vi "GaitDisplay.vi"() -> ()   [LabVIEW 2016]
uses:
  Classes/CAlex2-Display/CAlex2_Display.lvclass
  C:/Users/Rand/Documents/CAlex2-controller/Classes/CAlex2/CAlex2.lvclass
  C:/Users/Rand/Documents/CAlex2-controller/Classes/SerialChain/SerialChain.lvclass
  Classes/CAlex2/TypeDef/LowerBodyDim.ctl
  Classes/CAlex2/CAlex2.lvclass
  Classes/SerialChain/SerialChain.lvclass
panel:
  in  "port or service name":u16=11003
  in  "name":string="192.168.1.192"
  in  "Target":bool
  in  "Stop Button":bool
  in  "XY":bool
  in  "Reset":bool
  in  "Leg Position":refnum<k7>(container)
  # "Up"
  # "Back"
  # "Front"
  # "Down"
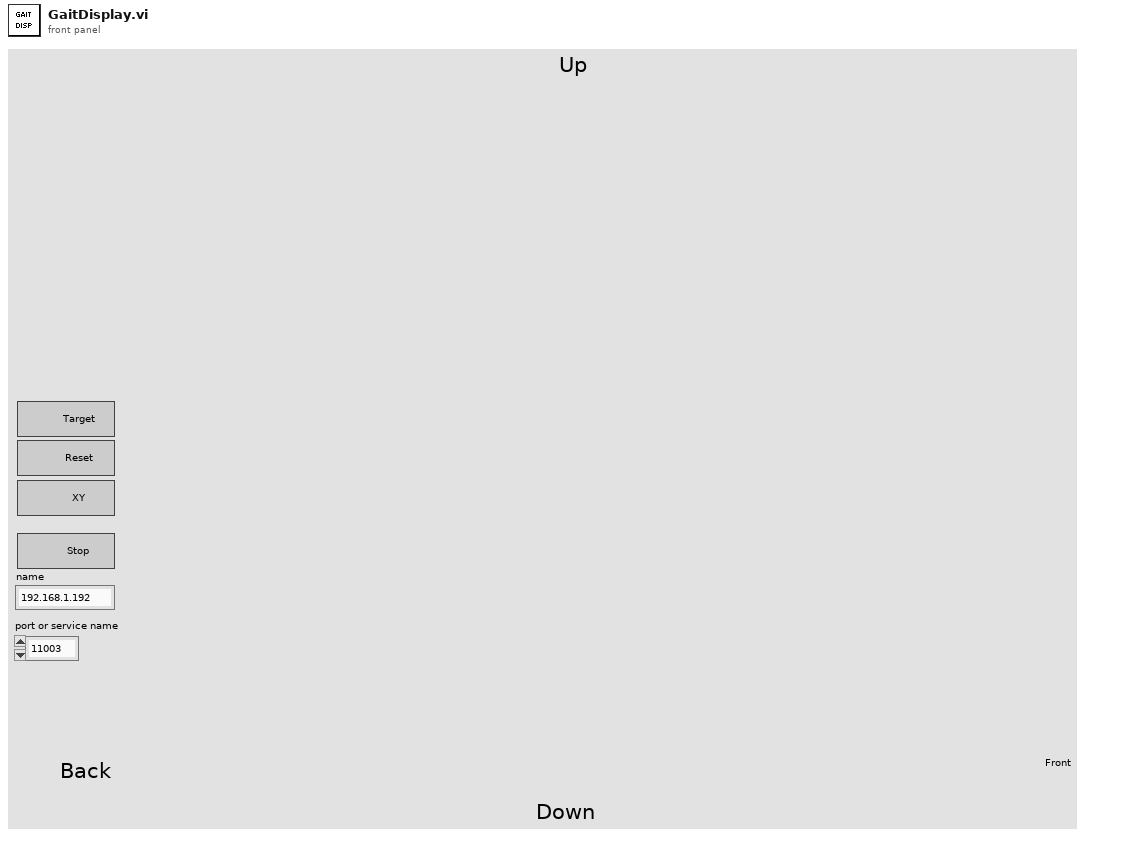
[diagram p1: front panel]
types:
  T1 = enum16{"big-endian, network order", "native, host order", "little-endian"}
  T2 = cluster{"AxisLabel":string[], "AxisMax":dbl[], "AxisMin":dbl[]}
  T3 = typedef "CAlex2.lvclass/LowerBodyDim.ctl" = cluster{"BodyDim":cluster{"ThighLt (m)":dbl, "ShankLt (m)":dbl, "HipWd (m)":dbl}, "BodyWt":cluster{"Thigh (kg)":dbl, "Shank (kg)":dbl}, "Cuff Loc":cluster{"HipCuffWd (m)":dbl, "HipCuffHt (m)":dbl, "HipFwdShift (m)":dbl, "ThighToKnee (m)":dbl, "ThighCuffDist (m)":dbl, "ShankToKnee (m)":dbl}}
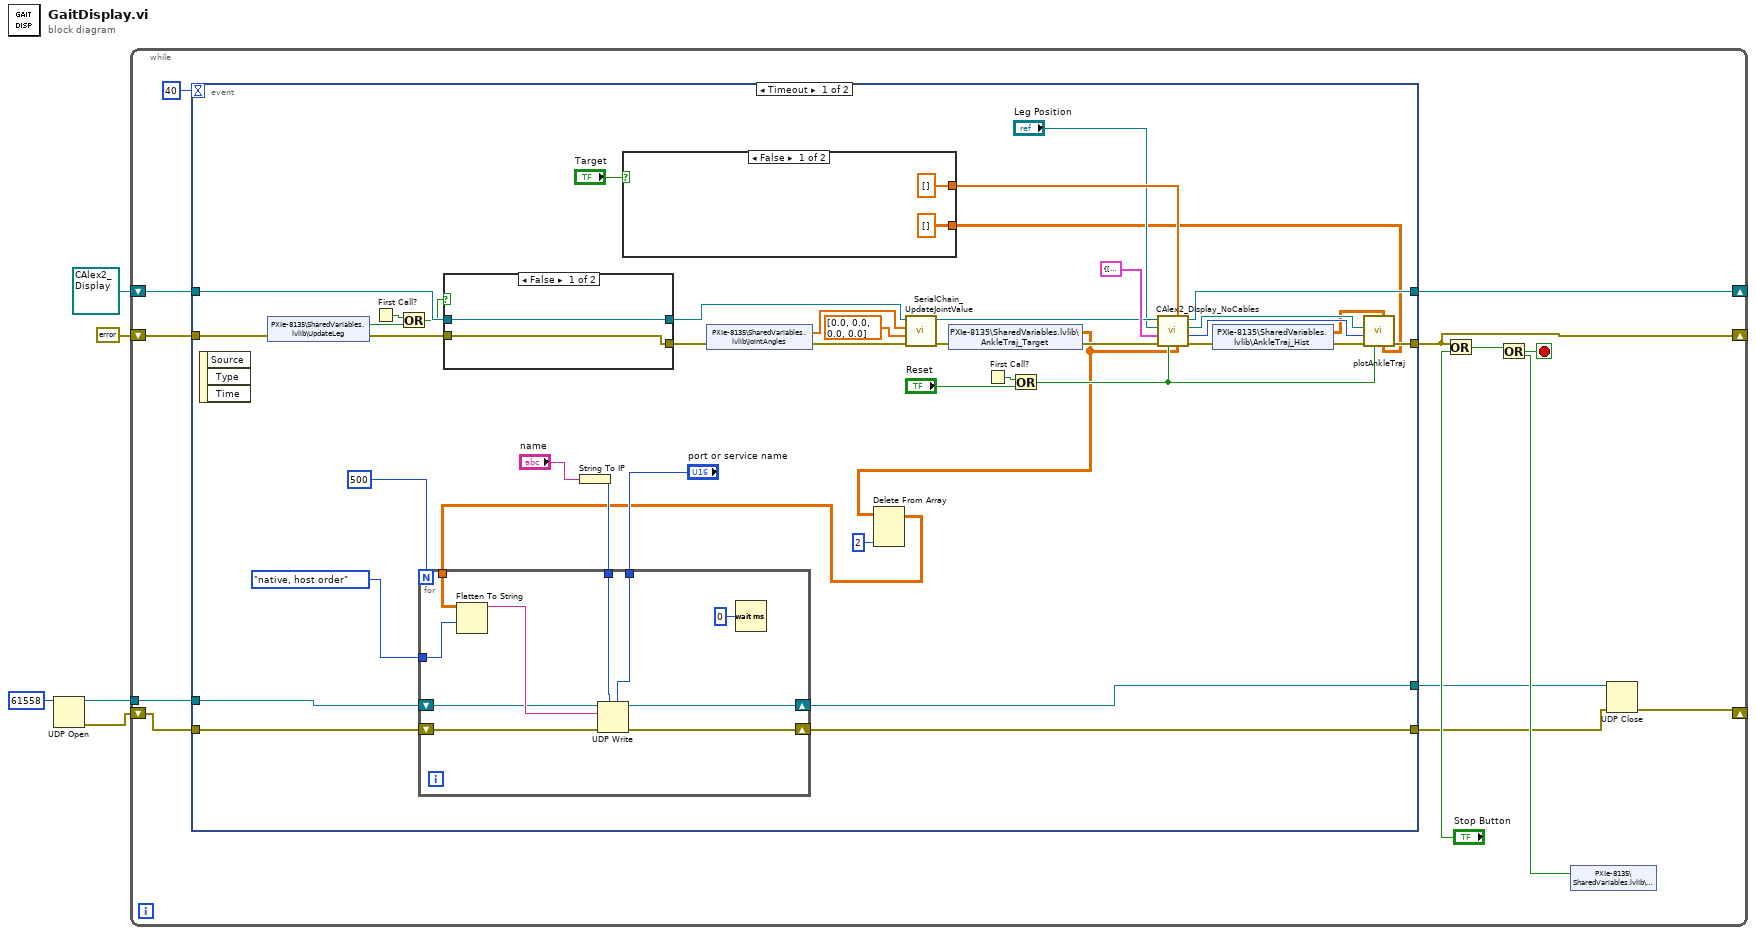
[diagram p0: block diagram]
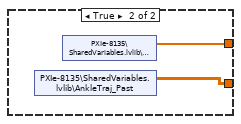
[diagram p2: hidden frame]
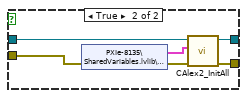
[diagram p3: hidden frame]
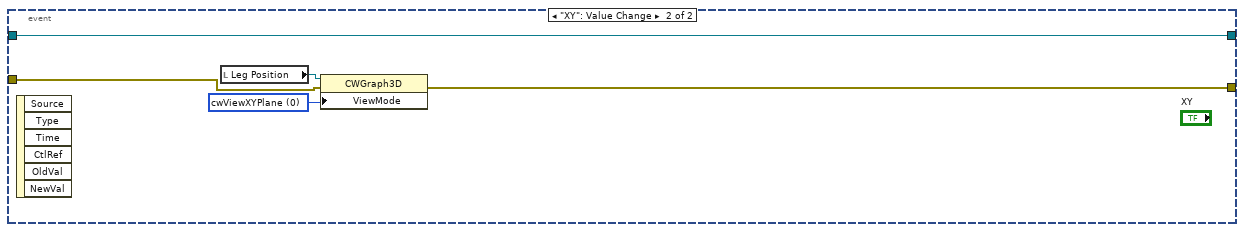
[diagram p4: hidden frame]
diagram:
  n1 = UDP Open(11:u16 61558 ("port")) -> (port=w1:refnum<k16>, 0:w3:errorcluster)  [unwired: 4 in, 1 out]
  n2 = while {
    shift-right: [w17] -> _
    shift-left: refnum<class "CAlex2_Display.lvclass"> refnum ("CAlex2") -> [w18]
    shift-right: [w15] -> _
    shift-left: errorcluster {"status"=FALSE, "code"=0, "source"=""} ("error out") -> [w11]
    shift-right: [w10] -> _
    shift-left: w3 -> [w9]
    tunnel: w1 -> [w7]
    stop <- w12 stop-if-true
    n3 = event shown="[0] Timeout" {
      selector: _ -> [_ _]
      dyn-events: _ -> [_ _]
      timeout: 40 -> [_ _]
      tunnel: w18 -> [w48 w83]
      tunnel: [w50 w83] -> w17
      tunnel: [w49 w85] -> w15
      tunnel: w11 -> [w45 w86]
      tunnel: w9 -> [w31 _]
      tunnel: [w26 _] -> w8
      tunnel: w7 -> [w25 _]
      tunnel: [w24 _] -> w6
      event Timeout {
        n4 = event-data() -> ()  [unwired: 1 in, 3 out]
        n5 = shared-variable "PXIe-8135\\SharedVariables.lvlib\\UpdateLeg"(error in=w45) -> (w41:bool, error out=w44:errorcluster)
        n6 = First Call?() -> (First Call?: T/F=w42:bool)
        n7 = Or(x=w42, y=w41) -> (x .or. y?=w40:bool)
        n8 = case shown="False" w40 {
          tunnel: w48 -> [w76 w82]
          tunnel: [w76 w81] -> w47
          tunnel: [w75 w78] -> w46
          tunnel: w44 -> [w75 w77]
          frame False {
          }
          frame True {
            n9 = shared-variable "PXIe-8135\\SharedVariables.lvlib\\LegDim"(error in=w77) -> (w80:T3, error out=w79:errorcluster)
            n10 = call "CAlex2_InitAll.vi"("error in (no error)"=w79, "LegProperties"=w80, "CAlex2 in"=w82) -> ("error out"=w78:errorcluster, "CAlex2 out"=w81:refnum<class "CAlex2_Display.lvclass">)  [unwired: 7 in]
          }
        }
        n11 = String To IP(1:"name") -> (0:w29:u32)
        n12 = case shown="False" "Target" {
          tunnel: [dbl[] [] ("Array of Double") w74] -> w55
          tunnel: [dbl[][] [] ("Array of Double") w73] -> w33
          frame False {
          }
          frame True {
            n13 = shared-variable "PXIe-8135\\SharedVariables.lvlib\\AnkleTraj_Past"() -> (w73:dbl[][])  [unwired: 1 in, 1 out]
            n14 = shared-variable "PXIe-8135\\SharedVariables.lvlib\\ClosestPt"() -> (w74:dbl[])  [unwired: 1 in, 1 out]
          }
        }
        n15 = shared-variable "PXIe-8135\\SharedVariables.lvlib\\JointAngles"(error in=w46) -> (w59:dbl[], error out=w58:errorcluster)
        n16 = call "SerialChain_UpdateJointValue.vi"("error in (no error)"=w58, "JointSpeed (rad/s | m/s)"=dbl[] [0.0, 0.0, 0.0, 0.0] ("JointSpeed (rad)"), "JointAngle (rad | m)"=w59, "SerialChain in"=w47) -> ("error out"=w32:errorcluster, "SerialChain out"=w51:refnum<class "CAlex2_Display.lvclass">)  [unwired: 6 in]
        n17 = shared-variable "PXIe-8135\\SharedVariables.lvlib\\AnkleTraj_Target"(error in=w32) -> (w27:dbl[][], error out=w34:errorcluster)
        n18 = Delete From Array(array=w27, index (col)=2 ("disabled index (col)")) -> (array with subset deleted=w21:dbl[][])  [unwired: 2 in, 1 out]
        n19 = for {
          N: 500 ("Numeric") -> [_]
          tunnel: w29 -> [w69]
          tunnel: "port or service name" -> [w68]
          tunnel: T1."native, host order" ("byte order (0:big-endian, network order)") -> [w63]
          tunnel: w21 -> [w62]
          shift-right: [w66] -> w26
          shift-left: w31 -> [w70]
          shift-right: [w64] -> w24
          shift-left: w25 -> [w65]
          n20 = Flatten To String(anything=w62, byte order (0:big-endian, network order)=w63) -> (data string=w67:string)  [unwired: 2 in, 2 out]
          n21 = UDP Write(address=w69, port or service name=w68, connection ID=w65, data in=w67, 8:w70) -> (error out=w66:errorcluster, 3:w64:refnum<k16>)  [unwired: 1 in]
          n22 = Wait (ms)(milliseconds to wait=u32 0) -> ()  [unwired: 1 out]
        }
        n23 = First Call?() -> (First Call?: T/F=w57:bool)
        n24 = Or(x=w57, y="Reset") -> (x .or. y?=w52:bool)
        n25 = call "CAlex2_Display_NoCables.vi"("AnkleTraj"=w27, "ClosePt"=w55, "Init?"=w52, "error in (no error)"=w34, "AxisSetting"=T2 {"AxisLabel"=["x ", "y", "z "], "AxisMax"=[0.75, 0.3, 0.8], "AxisMin"=[-0.75, -1.2, -0.7]}, "3D graph in"="Leg Position", "CLX2 in"=w51) -> ("error out"=w38:errorcluster, "LastPlotNum"=w53:i32, "3D graph out"=w54:refnum<k7>, "CLX2 out"=w50:refnum<class "CAlex2_Display.lvclass">)  [unwired: 1 in]
        n26 = shared-variable "PXIe-8135\\SharedVariables.lvlib\\AnkleTraj_Hist"(error in=w38) -> (w39:dbl[][], error out=w37:errorcluster)
        n27 = call "plotAnkleTraj.vi"("AnkleTraj_Prev"=w33, "AnkleTraj_history"=w39, "Init?"=w52, "error in (no error)"=w37, "PreviousPlotNum"=w53, "3D graph in"=w54) -> ("error out"=w49:errorcluster)  [unwired: 3 in, 2 out]
      }
      event "XY": Value Change {
        w87 = 0 items=["cwViewXYPlane", "cwViewXZPlane", "cwViewYZPlane", "cwViewUserDefined"] ("ViewMode")
        n28 = event-data() -> ()  [unwired: 1 in, 6 out]
        n29 = local read "Leg Position"() -> (w84:refnum<k7>)
        n30 = property class="CWGraph3D"(reference=w84, error in=w86, "ViewMode"=w87) -> (error out=w85:errorcluster)  [unwired: 1 out]
      }
    }
    n31 = Or(x=w15, y="Stop Button") -> (x .or. y?=w14:bool)
    n32 = shared-variable "PXIe-8135\\SharedVariables.lvlib\\Stop RT"() -> (w13:bool)  [unwired: 1 in, 1 out]
    n33 = Or(x=w14, y=w13) -> (x .or. y?=w12:bool)
    n34 = UDP Close(connection ID=w6, 8:w8) -> (error out=w10:errorcluster)  [unwired: 1 out]
  }
